vi "FTP Put and Get Files.vi"() -> ()   [LabVIEW 2019]
doc: "Demonstrates the use of the FTP VIs to \"put\" a binary file on an FTP server and \"get\" a text file from an FTP server."
uses:
  <vilib>/FTP/NI_FTP.lvlib
panel:
  out "Text in Retrieved File":string
  out "Retrieved File":path
  out "Sent File":path
  out "Data in Local File":dbl[](graph)
  # "Overview: Demonstrates the use of the FTP VIs to \"put\" a binary file on an FTP server and \"get\" a text file from an FTP server.\nInstructions:\nRun the VI."
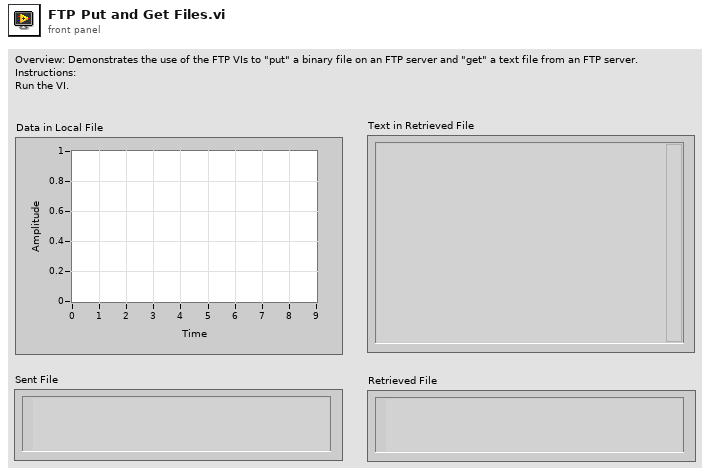
[diagram p1: front panel]
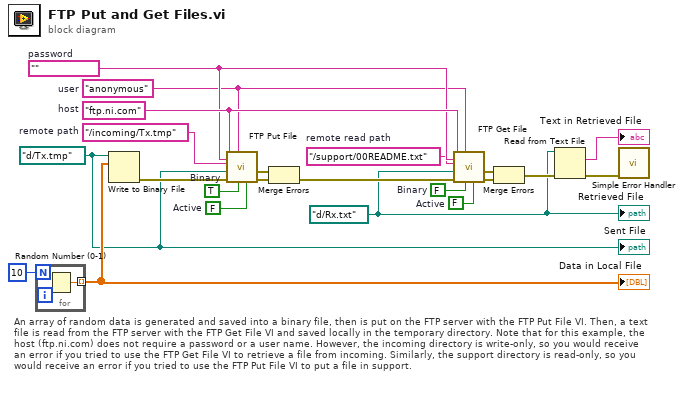
[diagram p0: block diagram]
diagram:
  w1 = FALSE  # Active
  w2 = FALSE  # Active
  w3 = "anonymous"  # user
  w4 = path "d:/Rx.txt" ("file (use dialog)")
  w7 = path "d:/Tx.tmp" ("file (use dialog)")
  w10 = FALSE  # Binary
  w9 = "/support/00README.txt"  # remote read path
  w11 = ""  # password
  w16 = TRUE  # Binary
  w17 = "/incoming/Tx.tmp"  # remote path
  w18 = "ftp.ni.com"  # host
  # "An array of random data is generated and saved into a binary file, then is put on the FTP server with the FTP Put File VI. Then, a text file is read from the FTP server with the FTP Get File VI and saved locally in the temporary directory. Note that for this example, the host (ftp.ni.com) does not require a password or a user name. However, the incoming directory is write-only, so you would receive an error if you tried to use the FTP Get File VI to retrieve a file from incoming. Similarly, the support directory is read-only, so you would receive an error if you tried to use the FTP Put File VI to put a file in support."
  n1 = for {
    N: 10 -> [_]
    tunnel: [w23] -> w21 mode=indexing
    n2 = Random Number (0-1)() -> (number: 0 to 1=w23:dbl)
  }
  "Data in Local File" <- w21
  n3 = Write to Binary File(file (use dialog)=w7, data=w21) -> (error out=w20:errorcluster)  [unwired: 4 in, 2 out]
  n4 = call <vilib>:"FTP Put File.vi"("active (T)"=w2, "password"=w11, "binary (F)"=w16, "user"=w3, "error in (no error)"=w20, "local path"=w7, "remote path"=w17, "host"=w18) -> ("error out"=w19:errorcluster, "file error"=w5:errorcluster)  [unwired: 2 in]
  n5 = Merge Errors(w5, w19) -> (w6:errorcluster)
  n6 = call <vilib>:"FTP Get File.vi"("active (T)"=w1, "password"=w11, "binary (F)"=w10, "user"=w3, "error in (no error)"=w6, "local path"=w4, "remote path"=w9, "host"=w18) -> ("error out"=w15:errorcluster, "file error"=w14:errorcluster)  [unwired: 2 in]
  n7 = Merge Errors(w14, w15) -> (w13:errorcluster)
  n8 = Read from Text File(file (use dialog)=w4, error in=w13) -> (text=→"Text in Retrieved File":string, error out=w12:errorcluster)  [unwired: 2 in, 2 out]
  n9 = call <vilib>:"Simple Error Handler.vi"("error in (no error)"=w12) -> ()  [unwired: 4 in, 5 out]
  "Sent File" <- w7
  "Retrieved File" <- w4
